vi "1WIRE_pulll_up_for_convert_multi.vi"(8 "error in":errorcluster) -> (0 "error out":errorcluster)   [LabVIEW 2016]
doc: "This VI is created by Vincent Claes for FPDA-1 more information on http://pwo.fpga.be\n\nvincent.claes@xios.be\nclaesvincent@gmail.com\n\nhttp://www.linkedin.com/in/vincentclaes"
uses:
  <vilib>/rvi/eio/common/nirviEmuTemplateMethod_errors.vi
  <vilib>/eio/EIONode/EIONode.xnode
  <vilib>/eio/EIOMethodNode/EIOMethodNode.xnode
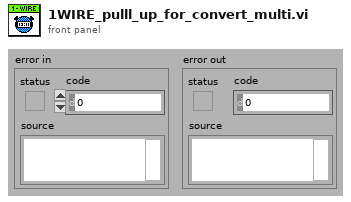
[diagram p1: front panel]
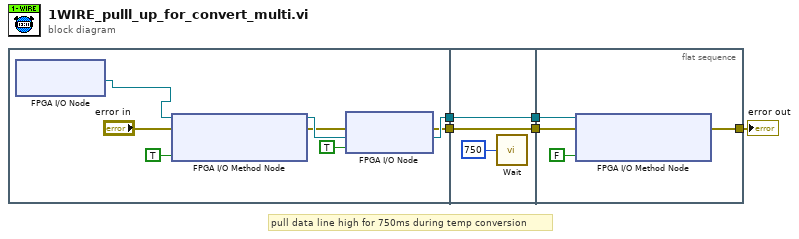
[diagram p0: block diagram]
diagram:
  # "pull data line high for 750ms during temp conversion"
  n1 = flat-sequence {
    tunnel: [w11] -> w5
    tunnel: [w8] -> w2
    tunnel: w5 -> [w15]
    tunnel: [w15] -> w4
    tunnel: [w14] -> w3
    tunnel: w2 -> [w14]
    tunnel: [w20] -> w1
    tunnel: w3 -> [w19]
    tunnel: w4 -> [w18]
    frame #0 {
      n2 = xnode "FPGA I/O Node"() -> ("FPGA I/O Out"=w6:refnum<k21>)  [unwired: 1 in, 1 out]
      n3 = xnode "FPGA I/O Method Node"("error in"="error in", "FPGA I/O In"=w6, "Enable"=TRUE) -> ("error out"=w9:errorcluster, "FPGA I/O Out"=w12:refnum<k21>)
      n4 = xnode "FPGA I/O Node"("error in"=w9, "I/O Item"=TRUE ("FX2_IO1_J1_0"), "FPGA I/O In"=w12) -> ("error out"=w8:errorcluster, "FPGA I/O Out"=w11:refnum<k21>)
    }
    frame #1 {
      n5 = call "Wait"("Count(mSec)"=u32 750 ("Count(uSec)")) -> ()  [unwired: 1 out]
    }
    frame #2 {
      n6 = xnode "FPGA I/O Method Node"("error in"=w19, "FPGA I/O In"=w18, "Enable"=FALSE) -> ("error out"=w20:errorcluster)  [unwired: 1 out]
    }
  }
  "error out" <- w1
